vi "Read Sound File to Graph.vi"() -> ()   [LabVIEW 2023]
doc: "This VI reads data from a sound file and plots it on a graph."
panel:
  out "File Data":waveform(dbl)[](graph)
  in  "Number of Samples":i32=-1
  out "Samples Read":i32
  # "Overview: Demonstrates the use of the Sound Functions to read data from a sound file and plot it on a graph.\nInstructions:\n1. Specify the Number of Samples to read (-1 for all).\n2. Run the VI. The waveform graph displays the specified number of samples from the sound file."
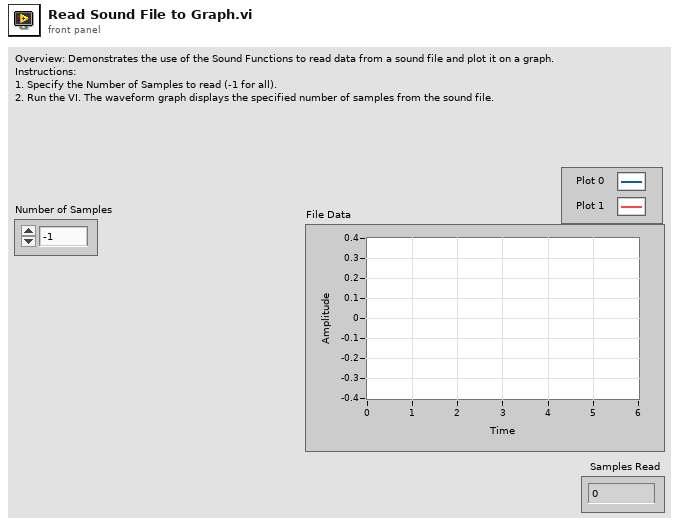
[diagram p1: front panel]
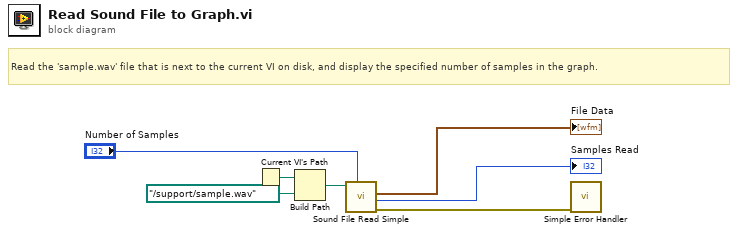
[diagram p0: block diagram]
diagram:
  # "Read the 'sample.wav' file that is next to the current VI on disk, and display the specified number of samples in the graph."
  n1 = Current VI's Path() -> (path=w1:path)
  n2 = Build Path(base path=w1, name or relative path=path "../support/sample.wav" ("Sound File Path")) -> (appended path=w2:path)
  n3 = call <vilib>:"Sound File Read Simple.vi"("number of samples/ch (-1: all)"="Number of Samples", "path"=w2) -> ("error out"=w4:errorcluster, "offset"=→"Samples Read":i32, "data"=→"File Data":waveform(dbl)[])  [unwired: 6 in, 1 out]
  n4 = call <vilib>:"Simple Error Handler.vi"("error in (no error)"=w4) -> ()  [unwired: 4 in, 5 out]
